vi "dfd_FIR Window Design.vi"(4 "param":dbl, 5 "window":u16(ring)=1 items=["None"=0, "Hanning"=1, "Hamming"=2, "Blackman-Harris"=3, "Exact Blackman"=4, "Blackman"=5, "Flat Top"=6, "4 Term B-Harris"=7, "7 Term B-Harris"=8, "Low Sidelobe"=9, "Triangular"=30, "Kaiser"=60, "Dolph-Chebyshev"=61, "Gaussian"=62], 6 "fs [Hz]":dbl=1.0, 7 "filter type":T1(ring), 8 "error in (no error)":errorcluster, 9 "low cutoff freq: fl":dbl=0.1, 10 "high cutoff freq: fh":dbl=0.3, 11 "order":i32=20) -> (0 "error out":errorcluster, 2 "h":dbl[](array[numeric]))   [LabVIEW 2017, in "NI_DigFilter_Design.lvlib"]
uses:
  <vilib>/addons/Digital Filter Design/NI_DigFilter_Design.lvlib
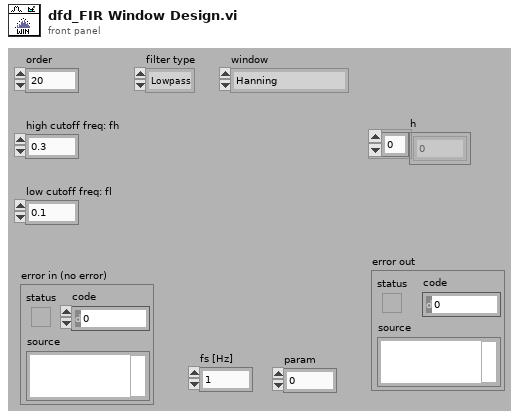
[diagram p1: front panel]
types:
  T1 = enum16{"Lowpass", "Highpass", "Bandpass", "Bandstop"}
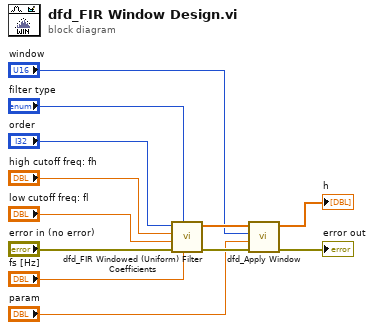
[diagram p0: block diagram]
diagram:
  n1 = call <vilib>:"dfd_FIR Windowed (Uniform) Filter Coefficients.vi"("sampling freq: fs"="fs [Hz]", "filter type"="filter type", "error in (no error)"="error in (no error)", "low cutoff freq: fl"="low cutoff freq: fl", "high cutoff freq: fh"="high cutoff freq: fh", "order"="order") -> ("error out"=w5:errorcluster, "FIR Coefficients"=w6:dbl[])  [unwired: 4 out]
  n2 = call <vilib>:"dfd_Apply Window.vi"("error in (no error)"=w5, "window param"="param", "window"="window", "x"=w6) -> ("error out"=→"error out":errorcluster, "windowed x"=→"h":dbl[])  [unwired: 6 out]
